vi "Teleop.vi"() -> ()   [LabVIEW 2020]
doc: "This VI is called for each TeleOp packet received from the DS where the robot is not disabled. It is often used to read from the joysticks and update I/O or to update setpoints for timed control loops. It should complete and return within 20 milliseconds or it may miss DS packets."
uses:
  <vilib>/Rock Robotics/WPI/Joystick/WPI_JoystickXBox Types.ctl
  <vilib>/Rock Robotics/WPI/Joystick/XBox Axes Indexer.ctl
  <vilib>/Rock Robotics/WPI/Joystick/XBox Buttons Indexer.ctl
  <vilib>/Rock Robotics/WPI/ThirdParty/REV Robotics/REVLib/Typedef/Spark MAX Sensor Type.ctl
  <vilib>/Rock Robotics/WPI/Utilities/WPI_GetSetVariantRefNum.vi
  Robot Global Data.vi
panel:
  in  "wallShoot":bool
  in  "padShoot":bool
  in  "Zero Intake":bool
  in  "High Shoot Button":bool
  in  "Low Shoot Button":bool
  in  "Spit Button":bool
  in  "Suck Button":bool
  in  "Shoot Button":bool
  in  "Joystick Deadband X":dbl=0.05
  in  "Joystick Deadband Y":dbl=0.05
  in  "Joystick 2 X Rotate":dbl(slide) scale=-1.0..1.0
  in  "Joystick 1 Y Forward/Back":dbl(slide) scale=1.0..-1.0
  in  "Joystick 1 X Strafe":dbl(slide) scale=-1.0..1.0
  in  "Override Joystick":bool
  in  "Joystick Deadband":dbl=0.05
  # "Assumptions to confirm coordinate systems:"
  # "Joystick Y Forward: -\nJoystick Y Back: +\n\nJoystick X Left: -\nJoystick X Right: +"
  # "Absolute Encoders:\nStraight Ahead 0\nLeft: (counterclockwise)  -180 or +180\nRight: (clockwise)  -180 or +180"
  # "Steering Encoders:\nLeft: (counterclockwise) - or +\nRight (clockwise) - or +"
  # "Manual Override Joysticks"
  # "Controls"
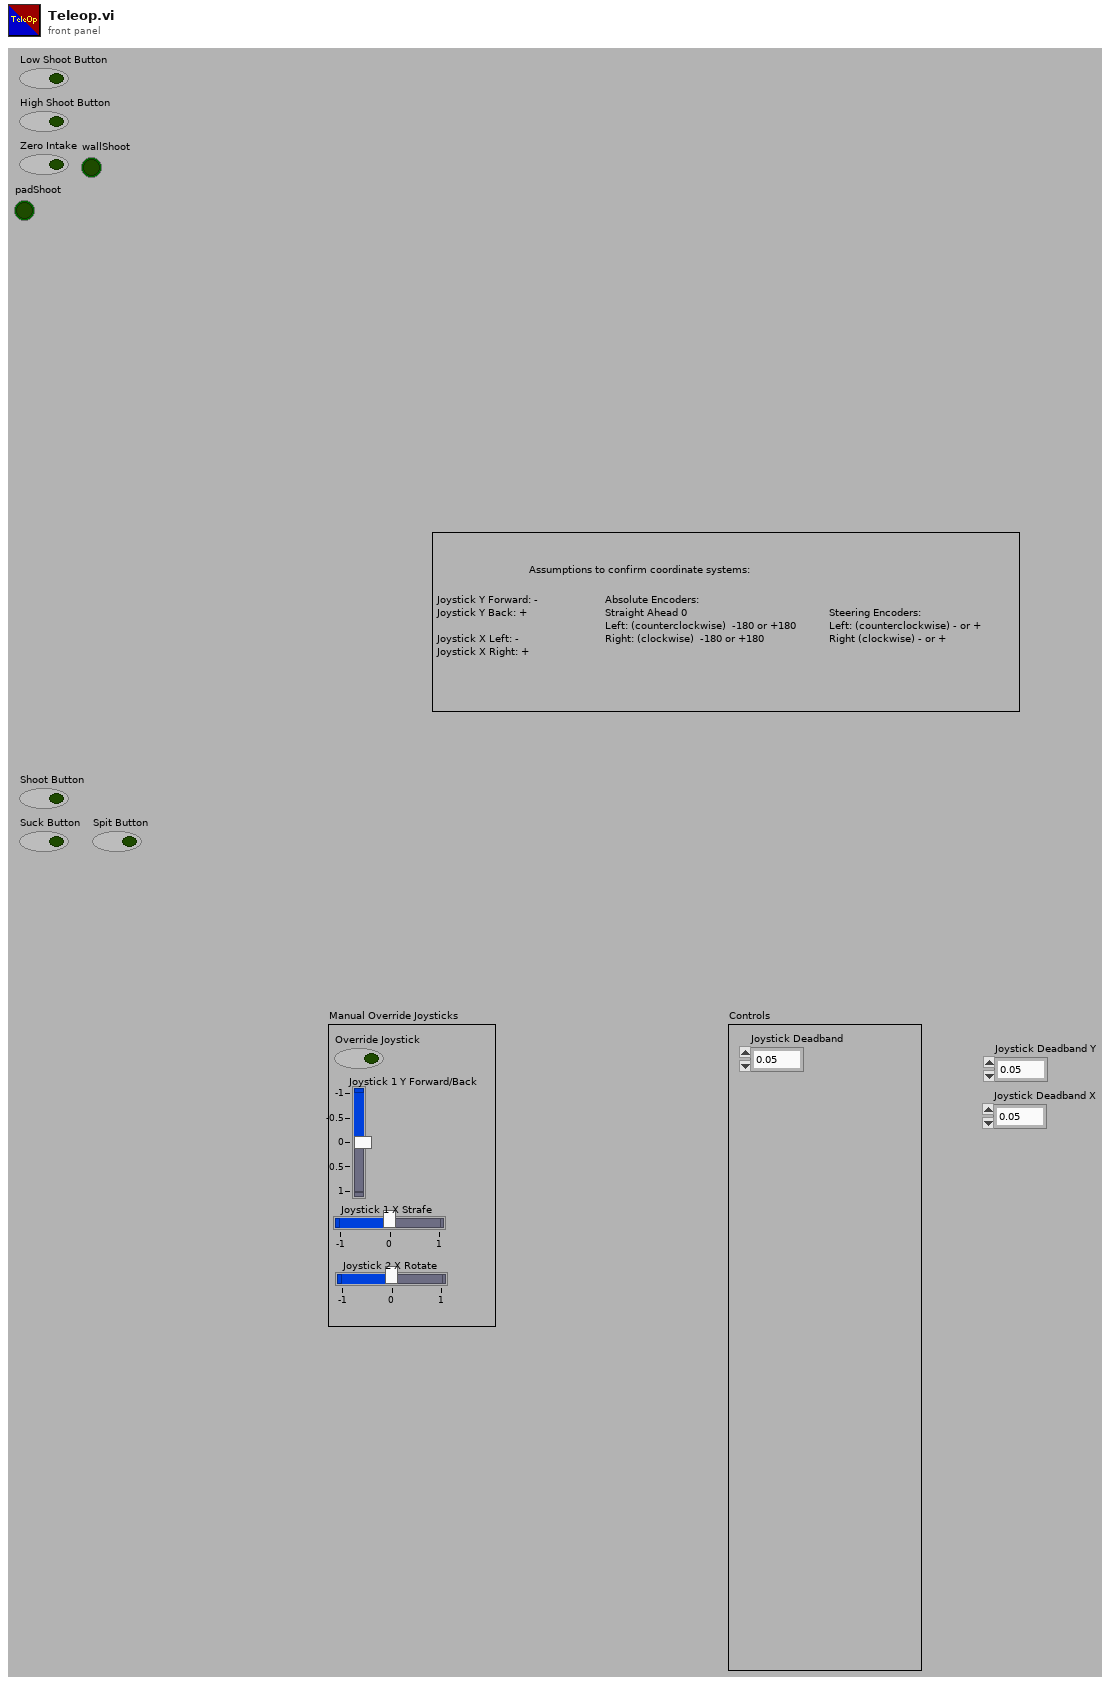
[diagram p1: front panel]
types:
  T1 = typedef "XBox Buttons Indexer.ctl" = enum16{"A", "B", "X", "Y", "Left Bumper", "Right Bumper", "Back", "Start", "Left Joystick", "Right Joystick"}
  T2 = typedef "XBox Axes Indexer.ctl" = enum16{"Left X", "Left Y", "Left Trigger", "Right Trigger", "Right X", "Right Y"}
  T3 = typedef "WPI_JoystickXBox Types.ctl" = enum16{"Not XBox", "XBox Unknown", "XBox Gamepad", "XBox Wheel", "XBox Arcade Stick", "XBox Flight Stick", "XBox Dance Pad", "XBox Guitar", "XBox Drum Kit", "XBox Arcade Pad"}
  T4 = typedef "WPI_JoystickDevRef.ctl" = cluster{"Device":T5}
  T5 = typedef "WPI_JoystickDeviceEnum.ctl" = enum16{"USB 0", "USB 1", "USB 2", "USB 3", "USB 4", "USB 5"}
  T6 = typedef "WPI_Joystick Info.ctl" = cluster{"Device Name":string, "HID Type":T7, "XBox Type":T3, "Axes Count":i32, "Axes Types":T8[], "Button Count":i32, "POV Count":i32}
  T7 = typedef "WPI_JoystickHID Types.ctl" = enum16{"Not HID", "HID Joystick", "HID Gamepad", "HID Driving Wheel", "HID Flightstick", "HID First Person"}
  T8 = typedef "WPI_JoystickAxis Types.ctl" = enum16{"X Axis", "Y Axis", "Z Axis", "RxAxis", "RyAxis", "RzAxis", "Slider", "POV", "None", "L X Axis", "L Y Axis", "L Trigger", "R Trigger", "R X Axis", "R Y Axis"}
  T9 = typedef "WPI_MotorControlDeviceRef.ctl" = cluster{"DeviceStatus":errorcluster, "Type":T10, "PWM":cluster{"PWM Channel":T11, "DeadBand":T12}, "CAN":cluster{"Device Number":u8, "SetOutput VI Ref":variant, "GetOutput VI Ref":variant, "Enable VI Ref":variant, "Disable VI Ref":variant, "Data":variant}, "Invert":bool, "DIO PWM":cluster{"PWM \"Enable\" Channel":T11, "DIOChannel":T13, "PWM Rate":dbl}}
  T10 = typedef "WPI_MotorControlType.ctl" = enum16{"PWM", "CAN", "DIO PWM"}
  T11 = typedef "FPGA_DIOPWMChannel.ctl" = enum8{"PWM 0", "PWM 1", "PWM 2", "PWM 3", "PWM 4", "PWM 5", "PWM 6", "PWM 7", "PWM 8", "PWM 9", "PWM MXP 0", "PWM MXP 1", "PWM MXP 2", "PWM MXP 3", "PWM MXP 4", "PWM MXP 5", "PWM MXP 6", "PWM MXP 7", "PWM MXP 8", "PWM MXP 9", "Invalid"}
  T12 = typedef "WPI_PWMDeadband.ctl" = cluster{"Name":string, "maxPositivePwm":i32, "minPositivePwm":i32, "centerPwm":i32, "maxNegativePwm":i32, "minNegativePwm":i32, "angularRange":u16}
  T13 = typedef "FPGA_DIOChannel.ctl" = enum8{"DIO 0", "DIO 1", "DIO 2", "DIO 3", "DIO 4", "DIO 5", "DIO 6", "DIO 7", "DIO 8", "DIO 9", "DIO MXP 0", "DIO MXP 1", "DIO MXP 2", "DIO MXP 3", "DIO MXP 4", "DIO MXP 5", "DIO MXP 6", "DIO MXP 7", "DIO MXP 8", "DIO MXP 9", "DIO MXP 10", "DIO MXP 11", "DIO MXP 12", "DIO MXP 13", "DIO MXP 14", "DIO MXP 15", "SPI Port CS1", "SPI Port CS2", "SPI Port CS3", "SPI Port MISO", "SPI Port MOSI", "Invalid"}
  T14 = typedef "Spark MAX Sensor Type.ctl" = enum16{"No Sensor", "Hall Sensor", "Encoder", "-Not Available-", "Analog", "Alternate Encoder"}
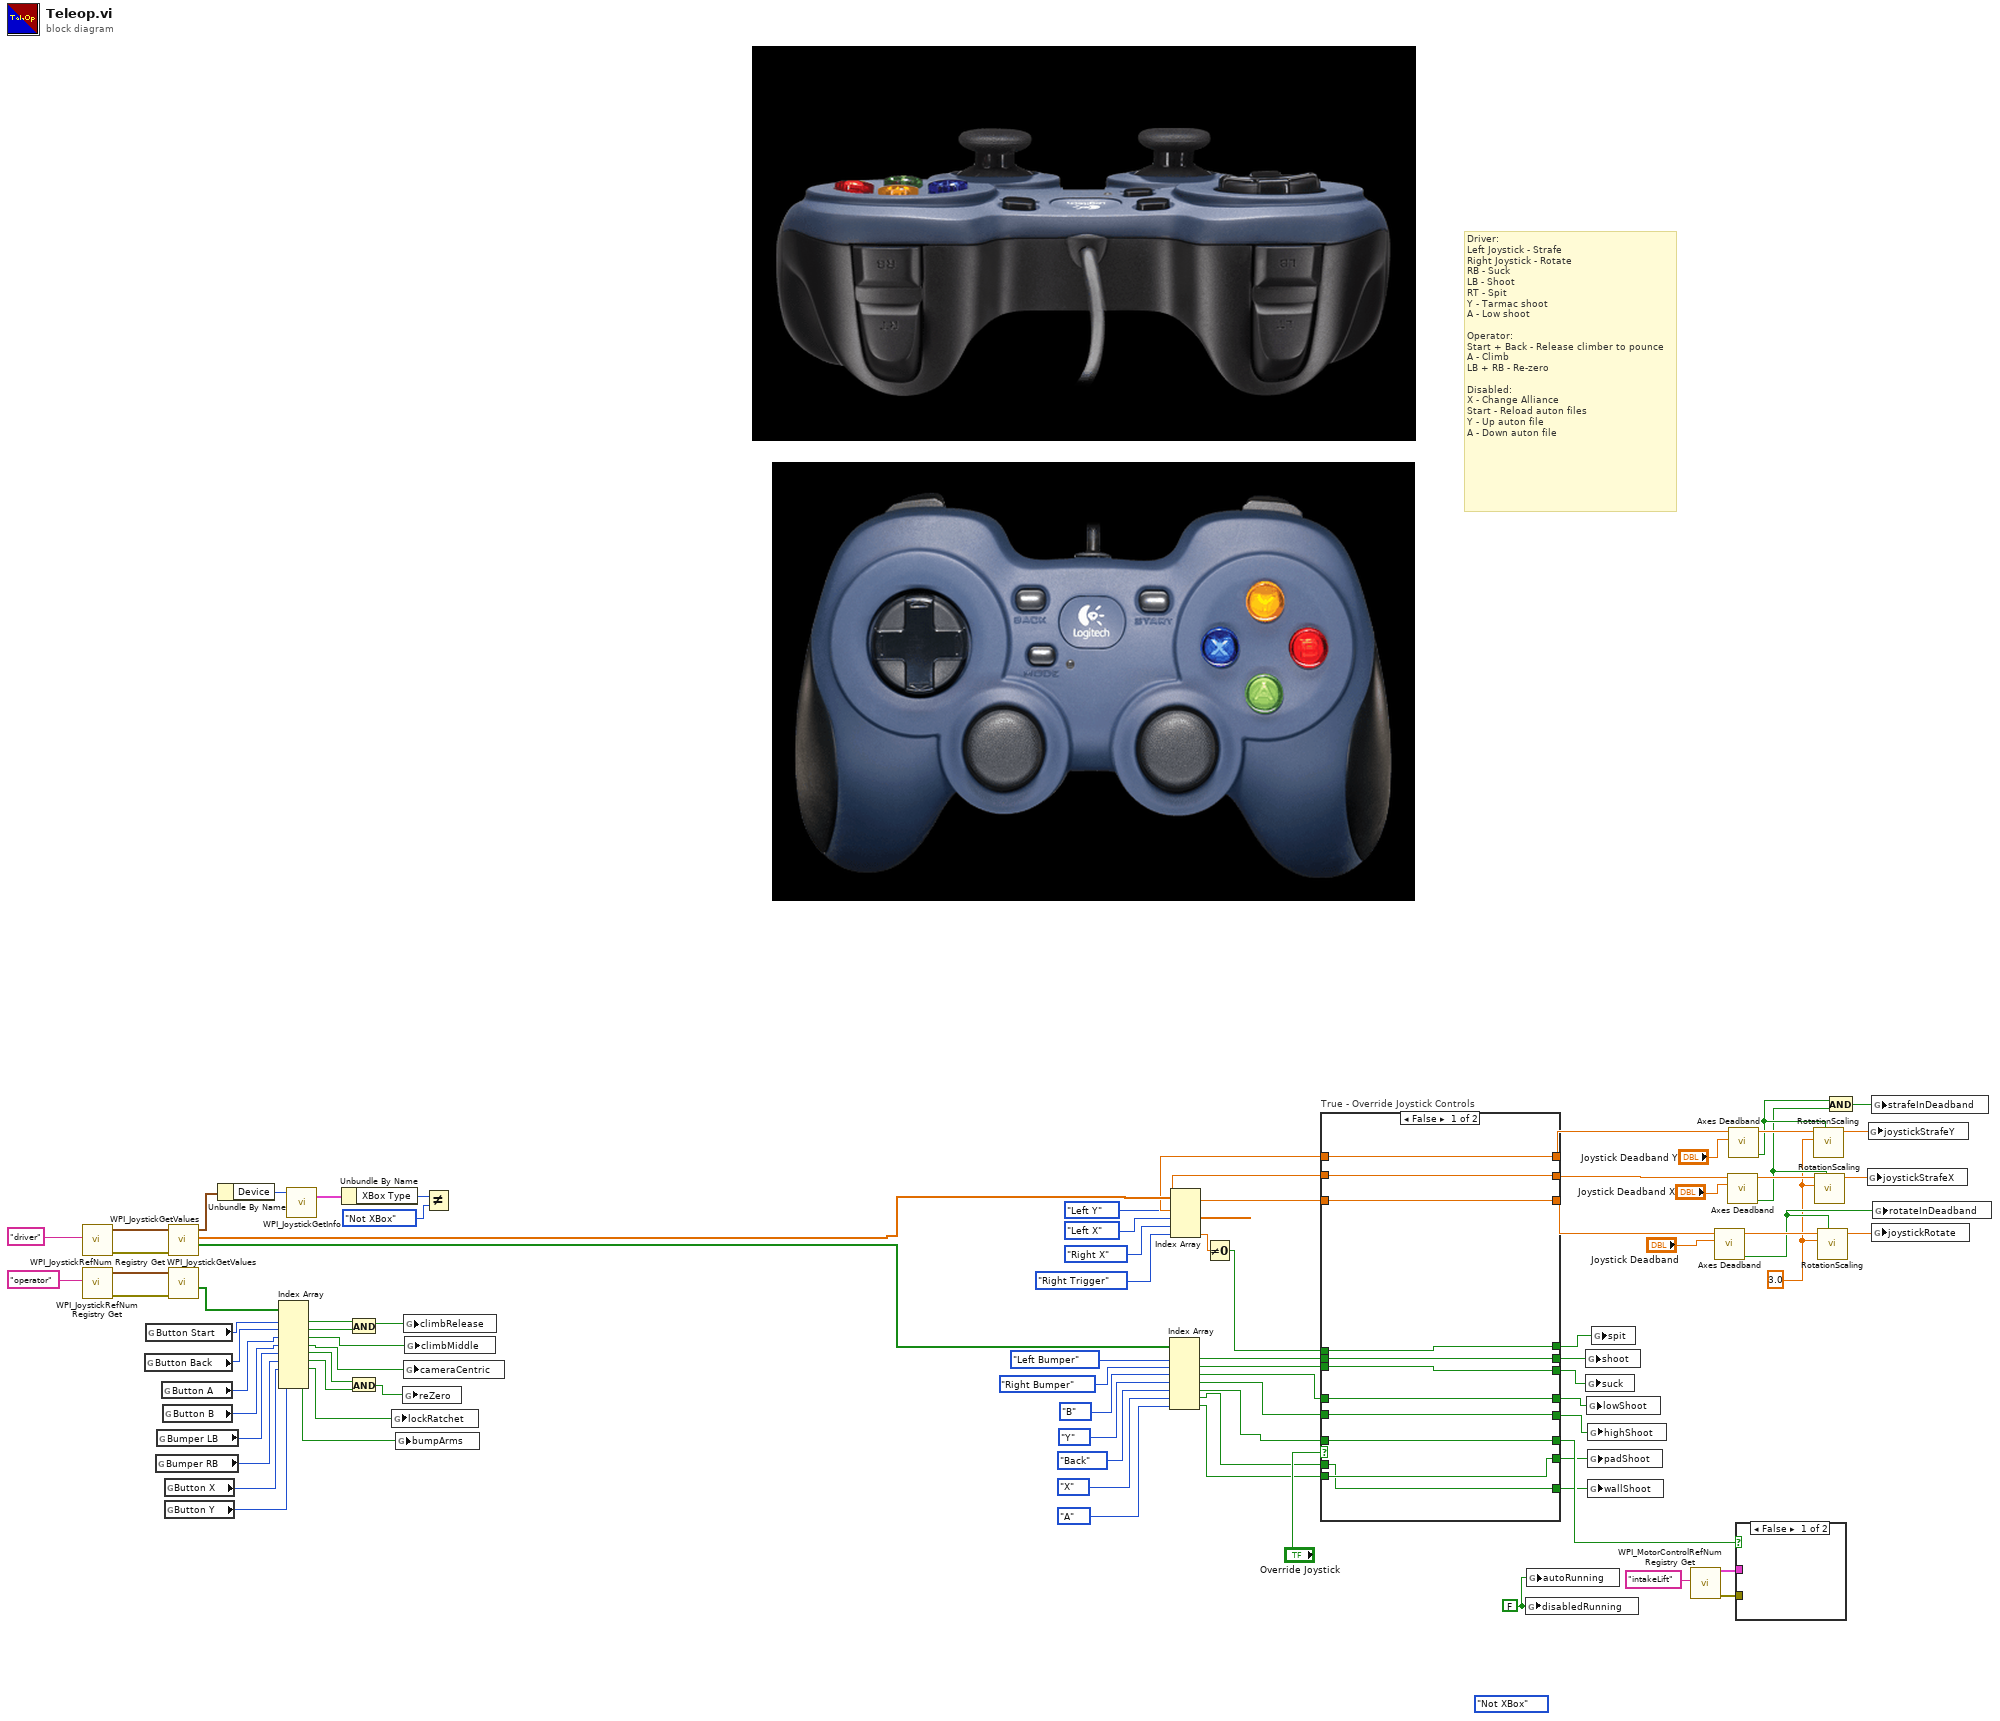
[diagram p0: block diagram]
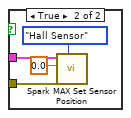
[diagram p2: hidden frame]
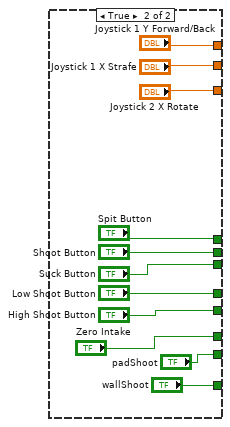
[diagram p3: hidden frame]
diagram:
  (unwired) WPI_JoystickXBox_Types."Not XBox" ("XBox Type")
  w61 = FALSE ("disabledRunning")
  w63 = 3.0 ("powerScale")
  # "Driver:\nLeft Joystick - Strafe\nRight Joystick - Rotate\nRB - Suck\nLB - Shoot\nRT - Spit\nY - Tarmac shoot\nA - Low shoot\n\nOperator:\nStart + Back - Release climber to pounce\nA - Climb\nLB + RB - Re-zero\n\nDisabled:\nX - Change Alliance\nStart - Reload auton files\nY - Up auton file\nA - Down auton file"
  n1 = call <vilib>:"WPI_JoystickRefNum Registry Get.vi"("refnum name"="driver") -> ("error out"=w80:errorcluster, "JoystickDevRef"=w58:T4)  [unwired: 9 in]
  n2 = call <vilib>:"WPI_JoystickRefNum Registry Get.vi"("refnum name"="operator") -> ("error out"=w79:errorcluster, "JoystickDevRef"=w78:T4)  [unwired: 9 in]
  n3 = global read "Robot Global Data.vi" "Button Back"() -> (w42:i32)
  n4 = global read "Robot Global Data.vi" "Button Start"() -> (w43:i32)
  n5 = global read "Robot Global Data.vi" "Bumper RB"() -> (w27:i32)
  n6 = global read "Robot Global Data.vi" "Bumper LB"() -> (w28:i32)
  n7 = global read "Robot Global Data.vi" "Button A"() -> (w38:i32)
  n8 = global read "Robot Global Data.vi" "Button B"() -> (w37:i32)
  n9 = global read "Robot Global Data.vi" "Button X"() -> (w25:i32)
  n10 = global read "Robot Global Data.vi" "Button Y"() -> (w18:i32)
  n11 = call <vilib>:"WPI_JoystickGetValues.vi"("error in (no error)"=w80, "JoystickDevRef"=w58) -> ("Buttons"=w51:bool[], "Axes"=w52:dbl[], "JoystickDevRef"=w56:T4)  [unwired: 5 in, 2 out]
  n12 = call <vilib>:"WPI_JoystickGetValues.vi"("error in (no error)"=w79, "JoystickDevRef"=w78) -> ("Buttons"=w44:bool[])  [unwired: 5 in, 4 out]
  n13 = Unbundle By Name(w56) -> ("Device"=w57:T5)
  n14 = Index Array(array=w44, index #1=w43, index #2=w42, index #3=w38, index #4=w37, index #5=w28, index #6=w27, index #7=w25, index #8=w18) -> (element #1=w41:bool, element #2=w40:bool, element #3=w36:bool, element #4=w31:bool, element #5=w30:bool, element #6=w29:bool, element #7=w24:bool, element #8=w17:bool)  [unwired: 1 in, 1 out]
  n15 = call <vilib>:"WPI_JoystickGetInfo.vi"("JoystickDevice"=w57) -> ("Joystick Info"=w55:T6)  [unwired: 9 in, 1 out]
  n16 = Unbundle By Name(w55) -> ("XBox Type"=w54:T3)
  n17 = And(x=w41, y=w40) -> (x .and. y?=w39:bool)
  n18 = And(x=w30, y=w29) -> (x .and. y?=w26:bool)
  n19 = global write "Robot Global Data.vi" "lockRatchet"(w24) -> ()
  n20 = global write "Robot Global Data.vi" "bumpArms"(w17) -> ()
  n21 = global write "Robot Global Data.vi" "reZero"(w26) -> ()
  n22 = global write "Robot Global Data.vi" "climbRelease"(w39) -> ()
  n23 = global write "Robot Global Data.vi" "cameraCentric"(w31) -> ()
  n24 = global write "Robot Global Data.vi" "climbMiddle"(w36) -> ()
  n25 = Not Equal?(x=w54, y=WPI_JoystickXBox_Types."Not XBox") -> ()  [unwired: 1 out]
  n26 = Index Array(array=w51, index #1=XBox_Buttons_Indexer."Left Bumper" ("XBox Buttons"), index #2=XBox_Buttons_Indexer."Right Bumper" ("XBox Buttons"), index #3=XBox_Buttons_Indexer."B" ("XBox Buttons"), index #4=XBox_Buttons_Indexer."Y" ("XBox Buttons"), index #5=XBox_Buttons_Indexer."Back" ("XBox Buttons"), index #6=XBox_Buttons_Indexer."X" ("XBox Buttons"), index #7=XBox_Buttons_Indexer."A" ("XBox Buttons")) -> (element #1=w46:bool, element #2=w45:bool, element #3=w35:bool, element #4=w32:bool, element #5=w23:bool, element #6=w4:bool, element #7=w3:bool)
  n27 = Index Array(array=w52, index #1=XBox_Axes_Indexer."Left Y" ("XBox Axes"), index #2=XBox_Axes_Indexer."Left X" ("XBox Axes"), index #3=XBox_Axes_Indexer."Right X" ("XBox Axes"), index #4=XBox_Axes_Indexer."Right Trigger" ("XBox Axes")) -> (element #1=w50:dbl, element #2=w49:dbl, element #3=w48:dbl, element #4=w12:dbl)
  n28 = Not Equal To 0?(x=w12) -> (x != 0?=w47:bool)
  n29 = case "True - Override Joystick Controls" shown="False" "Override Joystick" {
    tunnel: [w96 "Joystick 1 Y Forward/Back"] -> w77
    tunnel: [w94 "Joystick 2 X Rotate"] -> w83
    tunnel: [w95 "Joystick 1 X Strafe"] -> w74
    tunnel: [w92 "Shoot Button"] -> w62
    tunnel: [w91 "Suck Button"] -> w60
    tunnel: [w93 "Spit Button"] -> w59
    tunnel: w50 -> [w96 _]
    tunnel: w49 -> [w95 _]
    tunnel: w48 -> [w94 _]
    tunnel: w47 -> [w93 _]
    tunnel: w46 -> [w92 _]
    tunnel: w45 -> [w91 _]
    tunnel: w35 -> [w90 _]
    tunnel: [w90 "Low Shoot Button"] -> w34
    tunnel: [w89 "High Shoot Button"] -> w33
    tunnel: w32 -> [w89 _]
    tunnel: w23 -> [w88 _]
    tunnel: [w88 "Zero Intake"] -> w22
    tunnel: w4 -> [w86 _]
    tunnel: w3 -> [w87 _]
    tunnel: [w87 "padShoot"] -> w2
    tunnel: [w86 "wallShoot"] -> w1
    frame False {
    }
    frame True {
    }
  }
  n30 = global write "Robot Global Data.vi" "disabledRunning"(w61) -> ()
  n31 = global write "Robot Global Data.vi" "autoRunning"(w61) -> ()
  n32 = global write "Robot Global Data.vi" "shoot"(w62) -> ()
  n33 = global write "Robot Global Data.vi" "suck"(w60) -> ()
  n34 = global write "Robot Global Data.vi" "lowShoot"(w34) -> ()
  n35 = global write "Robot Global Data.vi" "highShoot"(w33) -> ()
  n36 = global write "Robot Global Data.vi" "padShoot"(w2) -> ()
  n37 = global write "Robot Global Data.vi" "wallShoot"(w1) -> ()
  n38 = global write "Robot Global Data.vi" "spit"(w59) -> ()
  n39 = call <vilib>:"WPI_MotorControlRefNum Registry Get.vi"("refnum name"="intakeLift") -> ("error out"=w19:errorcluster, "MotorControlDevRef"=w20:T9)  [unwired: 9 in]
  n40 = call "Axes Deadband.vi"("limit"="Joystick Deadband", "valueIn"=w83) -> ("inDeadband"=w64:bool, "valueOut"=w66:dbl)  [unwired: 8 in]
  n41 = call "Axes Deadband.vi"("limit"="Joystick Deadband X", "valueIn"=w74) -> ("inDeadband"=w67:bool, "valueOut"=w69:dbl)  [unwired: 8 in]
  n42 = call "Axes Deadband.vi"("limit"="Joystick Deadband Y", "valueIn"=w77) -> ("inDeadband"=w68:bool, "valueOut"=w70:dbl)  [unwired: 8 in]
  n43 = case shown="False" w22 {
    tunnel: w20 -> [_ w111]
    tunnel: w19 -> [_ w110]
    frame False {
    }
    frame True {
      n44 = call <vilib>:"Spark MAX Set Sensor Position.vi"("Sensor Type (Hall Sensor)"=Spark_MAX_Sensor_Type."Hall Sensor", "error in"=w110, "Position"=0.0, "MotorControlDeviceRef"=w111) -> ()  [unwired: 6 in, 2 out]
    }
  }
  n45 = call "RotationScaling.vi"("InDeadband"=w68, "powerScale"=w63, "Input"=w70) -> ("Output"=w72:dbl)  [unwired: 8 in]
  n46 = call "RotationScaling.vi"("InDeadband"=w67, "powerScale"=w63, "Input"=w69) -> ("Output"=w71:dbl)  [unwired: 8 in]
  n47 = call "RotationScaling.vi"("InDeadband"=w64, "powerScale"=w63, "Input"=w66) -> ("Output"=w65:dbl)  [unwired: 8 in]
  n48 = And(x=w68, y=w67) -> (x .and. y?=w73:bool)
  n49 = global write "Robot Global Data.vi" "joystickStrafeX"(w71) -> ()
  n50 = global write "Robot Global Data.vi" "joystickStrafeY"(w72) -> ()
  n51 = global write "Robot Global Data.vi" "strafeInDeadband"(w73) -> ()
  n52 = global write "Robot Global Data.vi" "joystickRotate"(w65) -> ()
  n53 = global write "Robot Global Data.vi" "rotateInDeadband"(w64) -> ()
